vi "VideoWriter Open_Default.vi"(4 "Fps":dbl=30.0, 5 "VideoCaptureAPIs":T1 items=["CAP_ANY"=0, "CAP_VFW/CAP_V4L"=200, "CAP_FIREWIRE"=300, "CAP_QT"=500, "CAP_UNICAP"=600, "CAP_DSHOW"=700, "CAP_PVAPI"=800, "CAP_OPENNI"=900, "CAP_OPENNI_ASUS"=910, "CAP_ANDROID"=1000, "CAP_XIAPI"=1100, "CAP_AVFOUNDATION"=1200, "CAP_GIGANETIX"=1300, "CAP_MSMF"=1400, "CAP_WINRT"=1410, "CAP_INTELPERC/CAP_REALSENSE"=1500, "CAP_OPENNI2"=1600, "CAP_OPENNI2_ASUS"=1610, "CAP_OPENNI2_ASTRA"=1620, "CAP_GPHOTO2"=1700, "CAP_GSTREAMER"=1800, "CAP_FFMPEG"=1900, "CAP_IMAGES"=2000, "CAP_ARAVIS"=2100, "CAP_OPENCV_MJPEG"=2200, "CAP_INTEL_MFX"=2300, "CAP_XINE"=2400, "CAP_UEYE"=2500, "CAP_OBSENSOR"=2600], 6 "FrameSize":T2, 7 "IsColor":bool, 8 "error in (no error)":errorcluster, 9 "Fourcc":string, 10 "Filename":string, 11 "VideoWriter in":refnum<class "VideoWriter.lvclass">) -> (0 "error out":errorcluster, 2 "Success":bool, 3 "VideoWriter out":refnum<class "VideoWriter.lvclass">)   [LabVIEW 2020, in "OpenLvVision_OpenCv.lvlib" / "VideoWriter.lvclass"]
doc: "Initializes or reinitializes video writer."
uses:
  VideoWriter.lvclass
  C:/Users/lukas/Downloads/OpenLvVision_OpenCv/SourceCode/LabView/OpenLvVision_OpenCv/_LvHelpers/EdvrObject/EdvrObject.lvclass
  TypeDef/Point/2D_PointI32.ctl
  TypeDef/VideoCaptureAPIs.ctl
  _LvHelpers/EdvrObject/EdvrObject.lvclass/EdvrObject.ctl
  OpenLvVision_OpenCv.lvlib
  _LvHelpers/EdvrObject/EdvrObject.lvclass
  Dlls/OlvOpenCvWrapper.dll
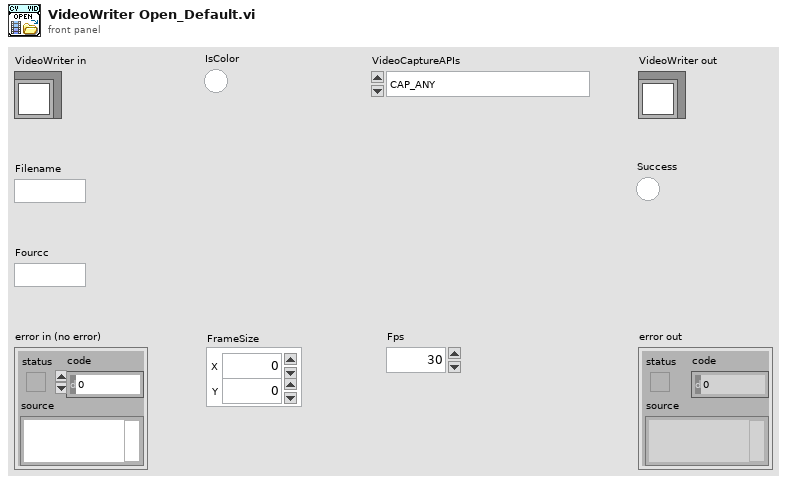
[diagram p1: front panel]
types:
  T1 = typedef "OpenLvVision_OpenCv.lvlib/VideoCaptureAPIs.ctl" = i32
  T2 = typedef "OpenLvVision_OpenCv.lvlib/2D_PointI32.ctl" = cluster{"X":i32, "Y":i32}
  T3 = typedef "OpenLvVision_OpenCv.lvlib/EdvrObject.lvclass/Edvr.ctl" = refnum<data-value>
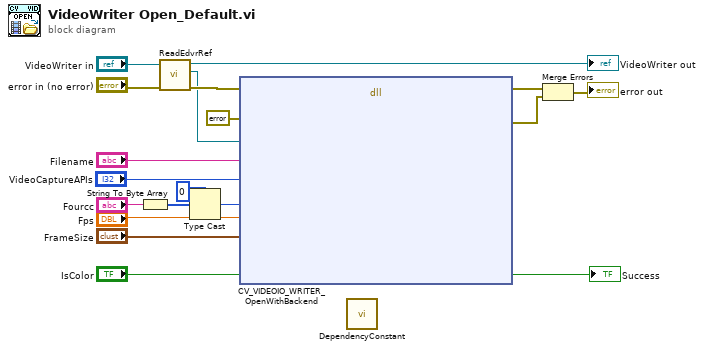
[diagram p0: block diagram]
diagram:
  n1 = String To Byte Array(string="Fourcc") -> (unsigned byte array=w6:u8[])
  n2 = call "ReadEdvrRef.vi"("error in (no error)"="error in (no error)", "EdvrObject in"="VideoWriter in") -> ("error out"=w18:errorcluster, "Edvr"=w17:T3, "EdvrObject out"=→"VideoWriter out":refnum<class "VideoWriter.lvclass">)  [unwired: 7 in]
  n3 = Type Cast(type=0, x=w6) -> (*(type *) &x=w5:i32)
  n4 = dll-call lib="C:/Users/lukas/Downloads/OpenLvVision_OpenCv/SourceCode/LabView/OpenLvVision_OpenCv/Dlls/OlvOpenCvWrapper.dll" fn="CV_VIDEOIO_WRITER_OpenWithBackend"(error in=w18, "Error"=errorcluster {"status"=FALSE, "code"=0, "source"=""} ("error out"), "edvrRef"=w17, "filename"="Filename", "apiPreference"="VideoCaptureAPIs", "fourcc"=w5, "fps"="Fps", "frameSize"="FrameSize", "isColor"="IsColor") -> (error out=w16:errorcluster, "Error"=w2:errorcluster, "Success"=→"Success":bool)  [unwired: 11 in, 1 out]
  n5 = call "DependencyConstant.vi"() -> ()  [unwired: 12 in]
  n6 = Merge Errors(w16, w2) -> (→"error out":errorcluster)
